vi "Wait_for_Temp.vi"(7 "LS336FrontPanel.vi":bool, 8 "error in (no error)":errorcluster, 10 "Message_command in":T1={"No. of command"=4, "Parameters"=["Within", "7", "A", "LS336", "30"], "Address"="GPIB0::12::INSTR", "Boolean"=TRUE, "No. of line"=448, "Initial Time"=timestamp(3623410447.312894 s since 1904-01-01), "Current Time"=timestamp(0 s since 1904-01-01), "Status"="Wait for Temperature Within than 7 K Sensor A of LS336 ( GPIB0::12::INSTR ) Timeout 30 min", "Sequence Ref."=refnum, "Temp check"=0, "Sequence_History"="", "Subsequence"=[]}, 11 "Command Queue":T2) -> (0 "error out":errorcluster, 2 "dup Message_command":T1={"No. of command"=4, "Parameters"=["Within", "7", "A", "LS336", "30"], "Address"="GPIB0::12::INSTR", "Boolean"=TRUE, "No. of line"=448, "Initial Time"=timestamp(3623410447.312894 s since 1904-01-01), "Current Time"=timestamp(0 s since 1904-01-01), "Status"="Wait for Temperature Within than 7 K Sensor A of LS336 ( GPIB0::12::INSTR ) Timeout 30 min\nCurrent Temperature : 7.9994 K\nElapsed Time : 2.9 min", "Sequence Ref."=refnum, "Temp check"=0, "Sequence_History"="", "Subsequence"=[]})   [LabVIEW 2019]
uses:
  Command_Queue.ctl
  Command_Message.ctl
panel:
  in  "timeout\nnotify?":bool=TRUE
  in  "within window":dbl=0.01
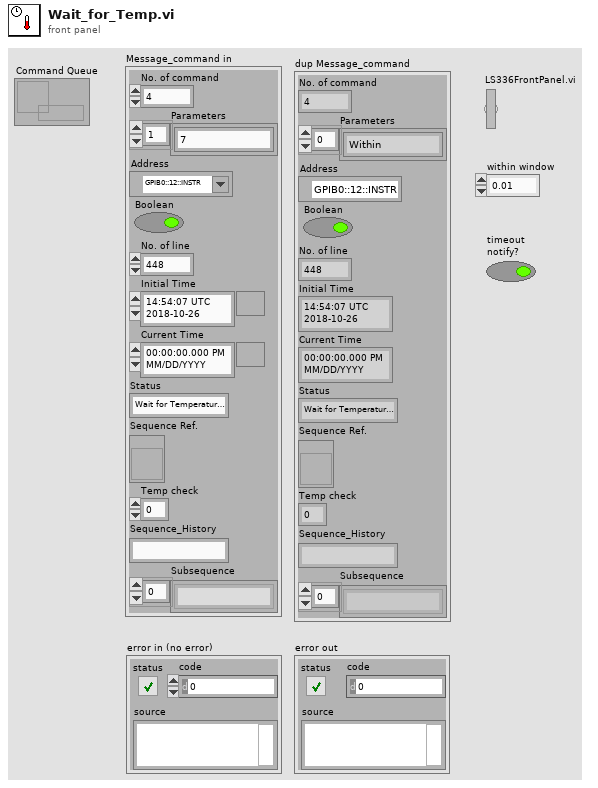
[diagram p1: front panel]
types:
  T1 = typedef "Command_Message.ctl" = cluster{"No. of command":i32, "Parameters":string[], "Address":refnum<visa-resource-name>, "Boolean":bool, "No. of line":i32, "Initial Time":timestamp, "Current Time":timestamp, "Status":string, "Sequence Ref.":refnum<vi>, "Temp check":i32, "Sequence_History":string, "Subsequence":string[]}
  T2 = typedef "Command_Queue.ctl" = refnum<queue>
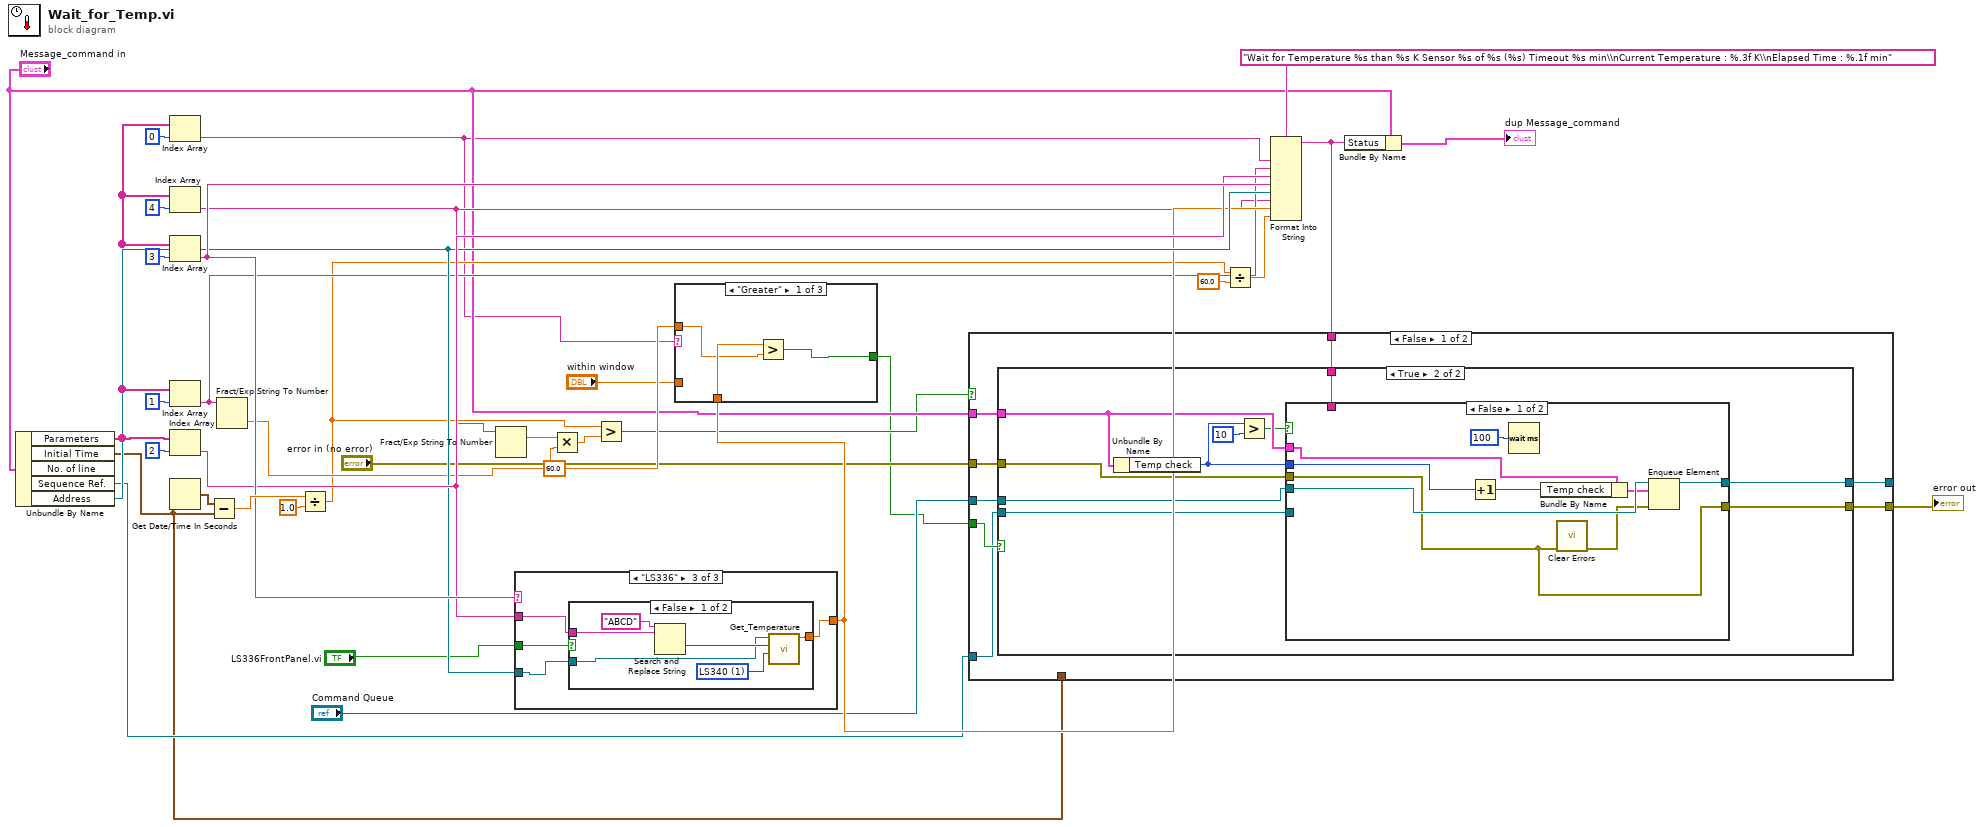
[diagram p0: block diagram]
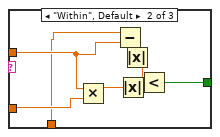
[diagram p2: hidden frame]
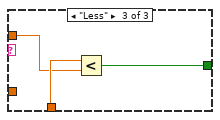
[diagram p3: hidden frame]
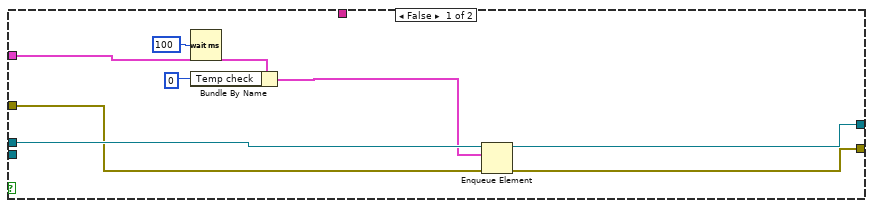
[diagram p4: hidden frame]
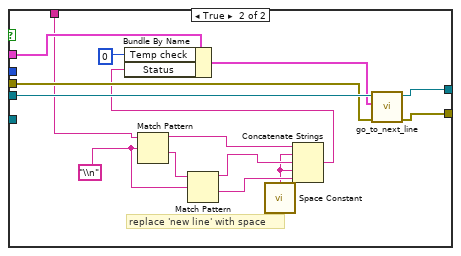
[diagram p5: hidden frame]
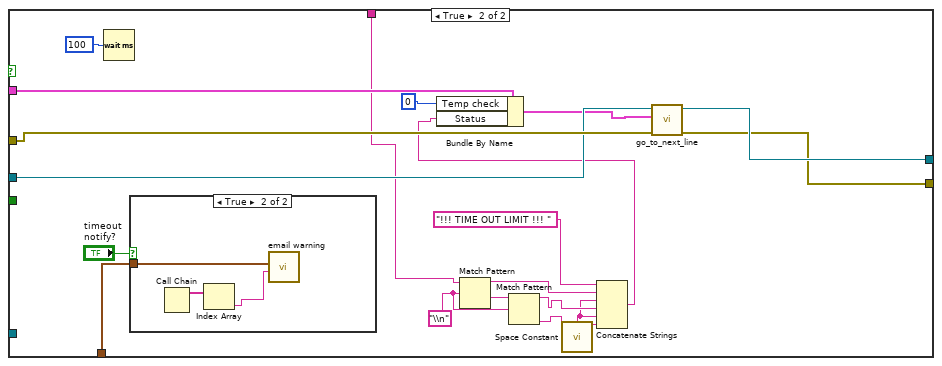
[diagram p6: hidden frame]
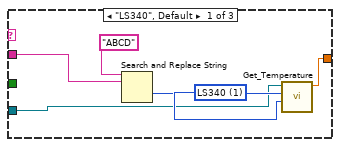
[diagram p8: hidden frame]
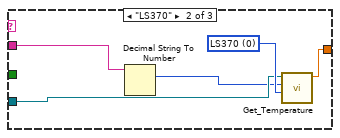
[diagram p9: hidden frame]
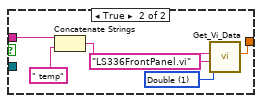
[diagram p10: hidden frame]
diagram:
  n1 = Unbundle By Name("Message_command in") -> ("Parameters"=w23:string[], "Initial Time"=w3:timestamp, "Sequence Ref."=w18:refnum<vi>, "Address"=w26:refnum<visa-resource-name>)  [unwired: 1 out]
  n2 = Index Array(array=w23, index=0) -> (element=w10:string)
  n3 = Index Array(array=w23, index=4) -> (element=w16:string)
  n4 = Index Array(array=w23, index=3) -> (element=w28:string)
  n5 = Index Array(array=w23, index=1) -> (element=w22:string)
  n6 = Index Array(array=w23, index=2) -> (element=w27:string)
  n7 = Get Date/Time In Seconds() -> (seconds since 1Jan1904=w24:timestamp)
  n8 = Subtract(x=w24, y=w3) -> (x-y=w30:dbl)
  n9 = Fract/Exp String To Number(string=w22) -> (number=w21:dbl)  [unwired: 3 in, 1 out]
  n10 = Divide(x=w30, y=1.0) -> (x/y=w13:dbl)
  n11 = Fract/Exp String To Number(string=w16) -> (number=w8:dbl)  [unwired: 3 in, 1 out]
  n12 = case shown="\"LS336\"" w28 {
    tunnel: w27 -> [w40 w44 w51]
    tunnel: w26 -> [w38 w46 w50]
    tunnel: [w37 w45 w49] -> w25
    tunnel: "LS336FrontPanel.vi" -> [_ _ w48]
    frame "LS340", Default {
      w42 = u16 1 items=["LS370", "LS340", "LS336"] ("Controller")
      n13 = Search and Replace String(input string="ABCD", search string=w40) -> (offset past replacement=w39:i32)  [unwired: 6 in, 3 out]
      n14 = call "Get_Temperature.vi"("Controller"=w42, "Channel"=w39, "VISA resource name"=w38) -> ("Temperature"=w37:dbl)  [unwired: 8 in]
    }
    frame "LS370" {
      w47 = u16 0 items=["LS370", "LS340", "LS336"] ("Controller")
      n15 = Decimal String To Number(string=w44) -> (number=w43:i32)  [unwired: 2 in, 1 out]
      n16 = call "Get_Temperature.vi"("Controller"=w47, "Channel"=w43, "VISA resource name"=w46) -> ("Temperature"=w45:dbl)  [unwired: 8 in]
    }
    frame "LS336" {
      n17 = case shown="False" w48 {
        tunnel: w51 -> [w52 w63]
        tunnel: [w53 w58] -> w49
        tunnel: w50 -> [w54 _]
        frame False {
          w55 = u16 1 items=["LS370", "LS340", "LS336"] ("Controller")
          n18 = Search and Replace String(input string="ABCD", search string=w52) -> (offset past replacement=w57:i32)  [unwired: 6 in, 3 out]
          n19 = call "Get_Temperature.vi"("Controller"=w55, "Channel"=w57, "VISA resource name"=w54) -> ("Temperature"=w53:dbl)  [unwired: 8 in]
        }
        frame True {
          w59 = u16 1 items=["String", "Double", "Boolean", "Variant"] ("Data Type")
          n20 = Concatenate Strings(w63, " temp" ("string")) -> (w61:string)
          n21 = call "Get_Vi_Data.vi"("Data Type"=w59, "VI name"="LS336FrontPanel.vi", "Control Name"=w61) -> ("Data (Double)"=w58:dbl)  [unwired: 4 in, 4 out]
        }
      }
    }
  }
  n22 = Multiply(x=w8, y=60.0) -> (x*y=w6:dbl)
  n23 = Greater?(x=w13, y=w6) -> (0:w9:bool)
  n24 = case shown="\"Greater\"" w10 {
    tunnel: w25 -> [w66 w67 w77]
    tunnel: w21 -> [w65 w70 w76]
    tunnel: [w64 w69 w75] -> w5
    tunnel: "within window" -> [_ w68 _]
    frame "Greater" {
      n25 = Greater?(x=w66, y=w65) -> (0:w64:bool)
    }
    frame "Within", Default {
      n26 = Multiply(x=w70, y=w68) -> (x*y=w72:dbl)
      n27 = Subtract(x=w67, y=w70) -> (x-y=w74:dbl)
      n28 = Absolute Value(x=w72) -> (abs(x)=w71:dbl)
      n29 = Absolute Value(x=w74) -> (abs(x)=w73:dbl)
      n30 = Less?(x=w73, y=w71) -> (x < y?=w69:bool)
    }
    frame "Less" {
      n31 = Less?(x=w77, y=w76) -> (x < y?=w75:bool)
    }
  }
  n32 = Divide(x=w13, y=60.0) -> (x/y=w14:dbl)
  n33 = Format Into String(format string="Wait for Temperature %s than %s K Sensor %s of %s (%s) Timeout %s min\\nCurrent Temperature : %.3f K\\nElapsed Time : %.1f min", w10, w22, w27, w28, w26, w16, w25, w14) -> (resulting string=w2:string)  [unwired: 2 in, 1 out]
  n34 = case shown="False" w9 {
    tunnel: w5 -> [w85 _]
    tunnel: "Message_command in" -> [w84 w140]
    tunnel: "Command Queue" -> [w83 w141]
    tunnel: "error in (no error)" -> [w82 w144]
    tunnel: w18 -> [w81 _]
    tunnel: [w80 w143] -> _
    tunnel: [w79 w142] -> w1
    tunnel: w3 -> [_ w139]
    tunnel: w2 -> [w78 w133]
    frame False {
      n35 = case shown="True" w85 {
        tunnel: w84 -> [w87 w101]
        tunnel: w83 -> [w93 w103]
        tunnel: w82 -> [w92 w102]
        tunnel: [w91 w96] -> w79
        tunnel: [w90 w97] -> w80
        tunnel: w81 -> [_ w95]
        tunnel: w78 -> [_ w94]
        frame False {
          n36 = Wait (ms)(milliseconds to wait=u32 100) -> ()  [unwired: 1 out]
          n37 = Bundle By Name(cluster=w87, "Temp check"=0) -> (w86:T1)
          n38 = Enqueue Element(queue=w93, element=w86, error in (no error)=w92) -> (queue out=w90:T2, error out=w91:errorcluster)  [unwired: 1 in, 1 out]
        }
        frame True {
          n39 = Unbundle By Name(w101) -> ("Temp check"=w98:i32)
          n40 = Greater?(x=w98, y=10) -> (0:w99:bool)
          n41 = case shown="False" w99 {
            tunnel: w103 -> [w112 w127]
            tunnel: w102 -> [w104 w126]
            tunnel: w101 -> [w110 w122]
            tunnel: w98 -> [w108 _]
            tunnel: [w107 w124] -> w97
            tunnel: [w104 w125] -> w96
            tunnel: w95 -> [_ _]
            tunnel: w94 -> [_ w117]
            frame False {
              n42 = Increment(x=w108) -> (x+1=w111:i32)
              n43 = Wait (ms)(milliseconds to wait=u32 100) -> ()  [unwired: 1 out]
              n44 = Bundle By Name(cluster=w110, "Temp check"=w111) -> (w109:T1)
              n45 = call <vilib>:"Clear Errors.vi"("error in (no error)"=w104) -> ("error out"=w105:errorcluster)  [unwired: 5 in, 1 out]
              n46 = Enqueue Element(queue=w112, element=w109, error in (no error)=w105) -> (queue out=w107:T2)  [unwired: 1 in, 2 out]
            }
            frame True {
              w120 = "\\n"
              # "replace 'new line' with space"
              n47 = Match Pattern(string=w117, regular expression=w120) -> (before substring=w119:string, after substring=w118:string)  [unwired: 1 in, 2 out]
              n48 = Match Pattern(string=w118, regular expression=w120) -> (before substring=w114:string, after substring=w115:string)  [unwired: 1 in, 2 out]
              n49 = call <vilib>:"Space Constant.vi"() -> ("String"=w113:string)
              n50 = Concatenate Strings(w119, w113, w114, w113, w115) -> (w116:string)
              n51 = Bundle By Name(cluster=w122, "Temp check"=0, "Status"=w116) -> (w121:T1)
              n52 = call "go_to_next_line.vi"("error in (no error)"=w126, "Message_command in"=w121, "Command Queue in"=w127) -> ("error out"=w125:errorcluster, "Command Queue out"=w124:T2)  [unwired: 7 in]
            }
          }
        }
      }
    }
    frame True {
      w137 = "\\n"
      n53 = Wait (ms)(milliseconds to wait=u32 100) -> ()  [unwired: 1 out]
      n54 = case shown="True" "timeout\nnotify?" {
        tunnel: w139 -> [_ w147]
        frame False {
        }
        frame True {
          n55 = Call Chain() -> (call chain=w149:string[])
          n56 = Index Array(array=w149) -> (element=w148:string)  [unwired: 1 in]
          n57 = call "email warning.vi"("running VI"=w148, "Initial"=w147) -> ()  [unwired: 9 in, 1 out]
        }
      }
      n58 = Match Pattern(string=w133, regular expression=w137) -> (before substring=w136:string, after substring=w135:string)  [unwired: 1 in, 2 out]
      n59 = Match Pattern(string=w135, regular expression=w137) -> (before substring=w129:string, after substring=w130:string)  [unwired: 1 in, 2 out]
      n60 = call <vilib>:"Space Constant.vi"() -> ("String"=w128:string)
      n61 = Concatenate Strings("!!! TIME OUT LIMIT !!! " ("string"), w136, w128, w129, w128, w130) -> (w131:string)
      n62 = Bundle By Name(cluster=w140, "Temp check"=0, "Status"=w131) -> (w132:T1)
      n63 = call "go_to_next_line.vi"("error in (no error)"=w144, "Message_command in"=w132, "Command Queue in"=w141) -> ("error out"=w142:errorcluster, "Command Queue out"=w143:T2)  [unwired: 7 in]
    }
  }
  "error out" <- w1
  n64 = Bundle By Name(cluster="Message_command in", "Status"=w2) -> (→"dup Message_command":T1)
